vi "Get GPS Data.vi"(8 "error in (no error)":errorcluster, 10 "sensor data":string, 11 "previous partial sentence":string) -> (0 "error out":errorcluster, 2 "GPS data":T1 {"oldest read timestamp" format="%^<%.3X\n%x>T"}, 3 "remaining partial sentence":string)   [LabVIEW 2011, in "u-blox 5 Series.lvlib"]
doc: "Parses <B>instrument data</B> in the NMEA format from GPS devices and returns common <B>GPS data</B>, such as the latitude and longitude of a fix."
uses:
  u-blox 5 Series.lvlib
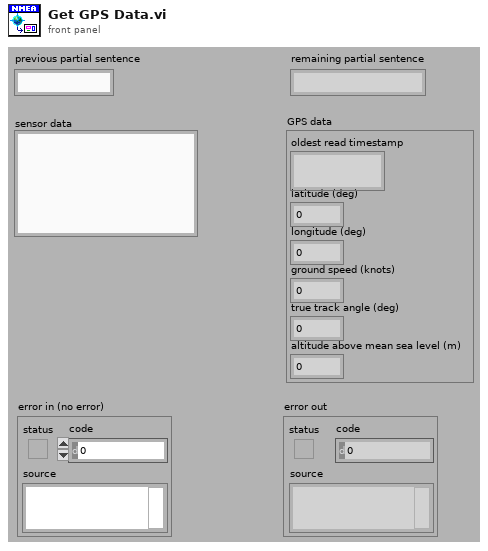
[diagram p1: front panel]
types:
  T1 = cluster{"oldest read timestamp":timestamp, "latitude (deg)":dbl, "longitude (deg)":dbl, "ground speed (knots)":dbl, "true track angle (deg)":dbl, "altitude above mean sea level (m)":dbl}
  T2 = cluster{"oldest read timestamp":timestamp, "latitude":dbl, "longitude":dbl, "speed over ground (knots)":dbl, "true track angle (deg)":dbl, "altitude above mean sea level":dbl}
  T3 = cluster{"Oldest Read Timestamp":timestamp, "Latitude":dbl, "Longitude":dbl, "Speed over Ground (Knots)":dbl, "True Track Angle (Deg)":dbl, "Altitude Above Mean Sea Level":dbl}
  T4 = typedef "u-blox 5 Series.lvlib/RMC Data.ctl" = cluster{"time of fix":cluster{"included?":bool, "time":timestamp}, "status":cluster{"included?":bool, "value":u16}, "latitude":cluster{"included?":bool, "latitude (deg)":dbl}, "longitude":cluster{"included?":bool, "longitude (deg)":dbl}, "ground speed":cluster{"included?":bool, "speed (knots)":dbl}, "true track angle":cluster{"included?":bool, "angle (deg)":dbl}, "magnetic variation":cluster{"included?":bool, "variation (deg)":dbl}, "type of fix":cluster{"included?":bool, "mode":u16}}
  T5 = typedef "u-blox 5 Series.lvlib/GGA Data.ctl" = cluster{"time of fix":cluster{"included?":bool, "time":timestamp}, "latitude":cluster{"included?":bool, "latitude (deg)":dbl}, "longitude":cluster{"included?":bool, "longitude (deg)":dbl}, "fix quality":cluster{"included?":bool, "quality":u16}, "number of satellites in view":cluster{"included?":bool, "number of satellites":i8}, "horizontal dilution of precision":cluster{"included?":bool, "horizontal DOP":dbl}, "altitude above mean sea level":cluster{"included?":bool, "altitude (m)":dbl}, "height of geoid above WGS84":cluster{"included?":bool, "height of geoid (m)":dbl}, "time since last DGPS update":cluster{"included?":bool, "time (s)":dbl}, "DGPS station ID number":cluster{"included?":bool, "station ID number":dbl}}
  T6 = typedef "u-blox 5 Series.lvlib/GLL Data.ctl" = cluster{"latitude":cluster{"included?":bool, "latitude (deg)":dbl}, "longitude":cluster{"included?":bool, "longitude (deg)":dbl}, "time of fix":cluster{"included?":bool, "time":timestamp}, "status":cluster{"included?":bool, "value":u16}, "type of fix":cluster{"included?":bool, "mode":u16}}
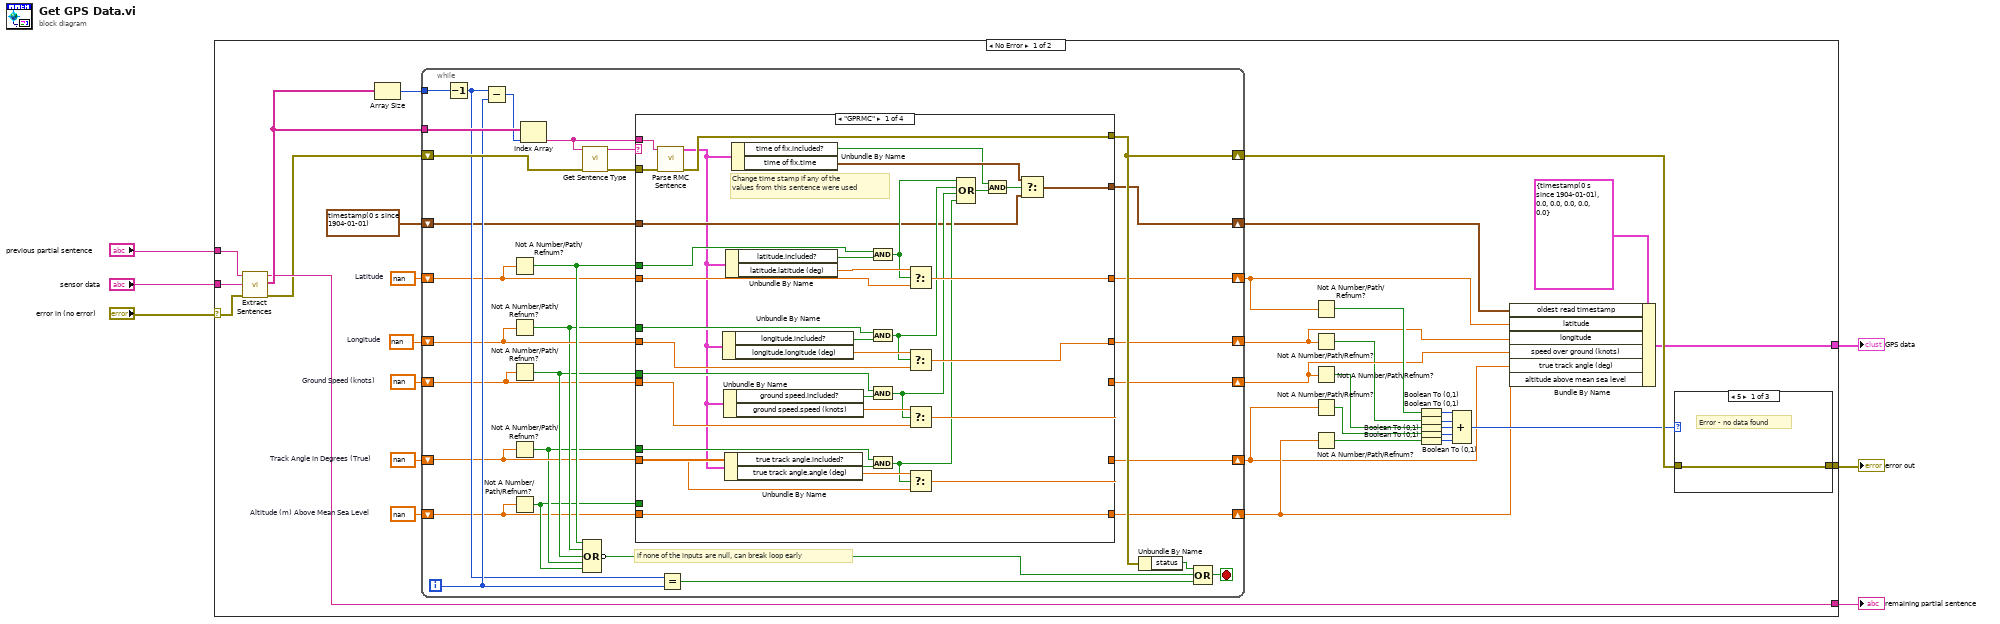
[diagram p0: block diagram]
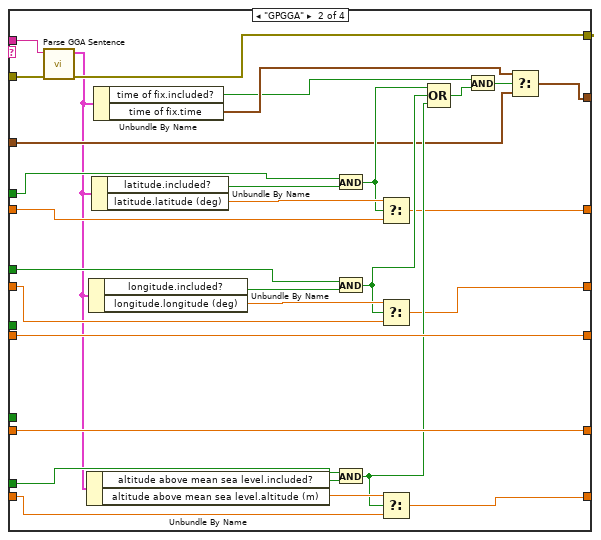
[diagram p4: hidden frame]
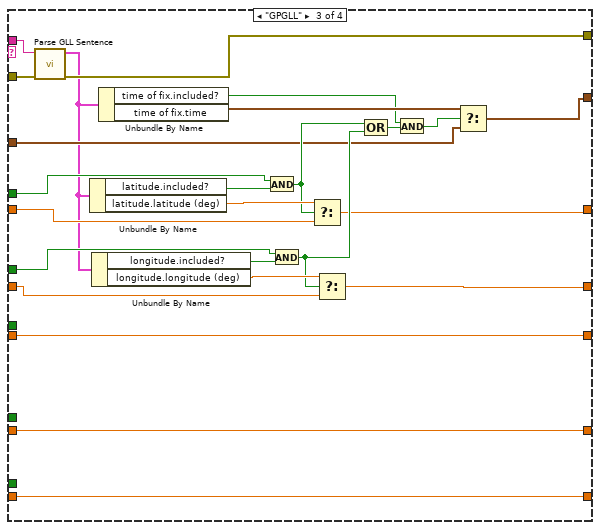
[diagram p5: hidden frame]
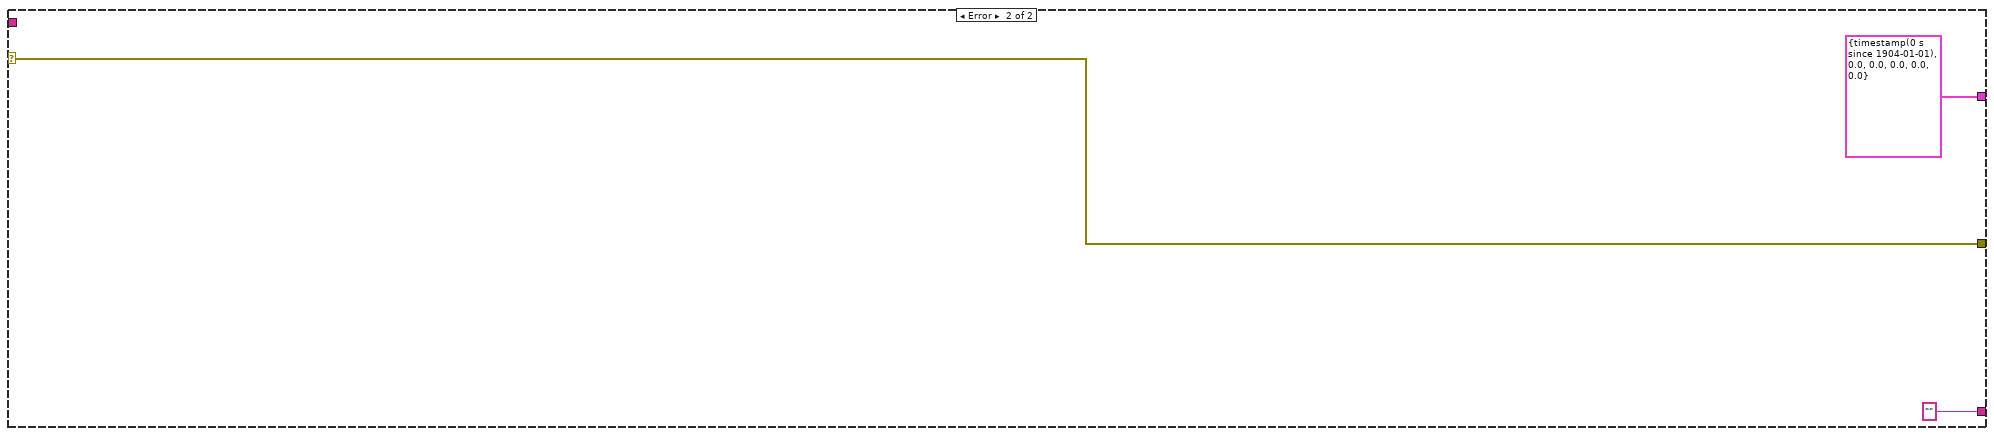
[diagram p7: hidden frame]
diagram:
  n1 = case shown="No Error" "error in (no error)" {
    selector: "error in (no error)" -> [w17 w174]
    tunnel: [w38 w174] -> w5
    tunnel: "sensor data" -> [w26 _]
    tunnel: "previous partial sentence" -> [w25 _]
    tunnel: [w24 T3 {"Oldest Read Timestamp"=timestamp(0 s since 1904-01-01), "Latitude"=0.0, "Longitude"=0.0, "Speed over Ground (Knots)"=0.0, "True Track Angle (Deg)"=0.0, "Altitude Above Mean Sea Level"=0.0} ("GPS Data")] -> w2
    tunnel: [w18 "" ("After Last Sentence")] -> w1
    frame No Error {
      w31 = nan  # Altitude (m) Above Mean Sea Level
      w32 = nan  # Track Angle in Degrees (True)
      w29 = nan  # Ground Speed (knots)
      w33 = nan  # Longitude
      w34 = nan  # Latitude
      n2 = call "Extract Sentences.vi"("error in (no error)"=w17, "sensor data"=w26, "previous partial sentence"=w25) -> ("error out"=w16:errorcluster, "complete sentences"=w37:string[], "remaining partial sentence"=w18:string)  [unwired: 4 in, 2 out]
      n3 = Array Size(array=w37) -> (size(s)=w36:i32)
      n4 = while {
        tunnel: w37 -> [w73]
        shift-right: [w69] -> w39
        shift-left: w16 -> [w71]
        shift-right: [w63] -> w40
        shift-left: timestamp(0 s since 1904-01-01) ("Time of Fix (UTC)") -> [w56]
        shift-right: [w61] -> w28
        shift-left: w34 -> [w54]
        shift-right: [w60] -> w11
        shift-left: w33 -> [w53]
        shift-right: [w68] -> w13
        shift-left: w32 -> [w49]
        shift-right: [w62] -> w14
        shift-left: w31 -> [w46]
        tunnel: w36 -> [w58]
        shift-right: [w59] -> w12
        shift-left: w29 -> [w50]
        i -> [w66]
        stop <- w74 stop-if-true
        # "if none of the inputs are null, can break loop early"
        n5 = Decrement(x=w58) -> (x-1=w57:i32)
        n6 = Subtract(x=w57, y=w66) -> (x-y=w67:i32)
        n7 = Not A Number/Path/Refnum?(number/path/refnum=w54) -> (NaN/Path/Refnum?=w55:bool)
        n8 = Not A Number/Path/Refnum?(number/path/refnum=w53) -> (NaN/Path/Refnum?=w52:bool)
        n9 = Not A Number/Path/Refnum?(number/path/refnum=w50) -> (NaN/Path/Refnum?=w51:bool)
        n10 = Not A Number/Path/Refnum?(number/path/refnum=w49) -> (NaN/Path/Refnum?=w48:bool)
        n11 = Not A Number/Path/Refnum?(number/path/refnum=w46) -> (NaN/Path/Refnum?=w47:bool)
        n12 = Index Array(array=w73, index=w67) -> (element=w45:string)
        n13 = call "Get Sentence Type.vi"("error in (no error)"=w71, "sentence"=w45) -> ("error out"=w70:errorcluster, "sentence type"=w44:string)  [unwired: 1 in, 7 out]
        n14 = Compound Arithmetic op=OR(w55, w52, w51, w48, w47) -> (invert w64:bool)
        n15 = case shown="\"GPRMC\"" w44 {
          tunnel: w70 -> [w109 w139 w164 w171]
          tunnel: [w108 w137 w162 w171] -> w69
          tunnel: [w102 w138 w163 w170] -> w68
          tunnel: w45 -> [w76 w111 w141 _]
          tunnel: w56 -> [w81 w114 w143 w169]
          tunnel: w54 -> [w88 w119 w150 w167]
          tunnel: w53 -> [w93 w125 w156 w166]
          tunnel: w49 -> [w103 w138 w163 w170]
          tunnel: w46 -> [w107 w133 w161 w168]
          tunnel: w55 -> [w90 w120 w151 _]
          tunnel: w52 -> [w95 w127 w152 _]
          tunnel: w51 -> [w97 _ _ _]
          tunnel: w48 -> [w105 _ _ _]
          tunnel: w47 -> [_ w132 _ _]
          tunnel: [w77 w113 w142 w169] -> w63
          tunnel: [w107 w130 w161 w168] -> w62
          tunnel: [w87 w121 w149 w167] -> w61
          tunnel: [w98 w136 w160 w165] -> w59
          tunnel: [w92 w124 w155 w166] -> w60
          tunnel: w50 -> [w99 w136 w160 w165]
          frame "GPRMC" {
            # "Change time stamp if any of the\nvalues from this sentence were used"
            n16 = call "Parse RMC Sentence.vi"("error in (no error)"=w109, "RMC sentence"=w76) -> ("error out"=w108:errorcluster, "RMC data"=w75:T4)  [unwired: 8 in]
            n17 = Unbundle By Name(w75) -> ("longitude.included?"=w96:bool, "longitude.longitude (deg)"=w94:dbl)
            n18 = Unbundle By Name(w75) -> ("ground speed.included?"=w101:bool, "ground speed.speed (knots)"=w100:dbl)
            n19 = Unbundle By Name(w75) -> ("true track angle.included?"=w106:bool, "true track angle.angle (deg)"=w104:dbl)
            n20 = Unbundle By Name(w75) -> ("latitude.included?"=w91:bool, "latitude.latitude (deg)"=w89:dbl)
            n21 = Unbundle By Name(w75) -> ("time of fix.included?"=w79:bool, "time of fix.time"=w80:timestamp)
            n22 = And(x=w90, y=w91) -> (x .and. y?=w86:bool)
            n23 = And(x=w95, y=w96) -> (x .and. y?=w85:bool)
            n24 = And(x=w97, y=w101) -> (x .and. y?=w84:bool)
            n25 = And(x=w105, y=w106) -> (x .and. y?=w83:bool)
            n26 = Select(t=w89, s=w86, f=w88) -> (s? t:f=w87:dbl)
            n27 = Select(t=w94, s=w85, f=w93) -> (s? t:f=w92:dbl)
            n28 = Select(t=w100, s=w84, f=w99) -> (s? t:f=w98:dbl)
            n29 = Select(t=w104, s=w83, f=w103) -> (s? t:f=w102:dbl)
            n30 = Compound Arithmetic op=OR(w86, w85, w84, w83) -> (w82:bool)
            n31 = And(x=w79, y=w82) -> (x .and. y?=w78:bool)
            n32 = Select(t=w80, s=w78, f=w81) -> (s? t:f=w77:timestamp)
          }
          frame "GPGGA" {
            n33 = call "Parse GGA Sentence.vi"("error in (no error)"=w139, "GGA sentence"=w111) -> ("error out"=w137:errorcluster, "GGA data"=w110:T5)  [unwired: 8 in]
            n34 = Unbundle By Name(w110) -> ("altitude above mean sea level.included?"=w135:bool, "altitude above mean sea level.altitude (m)"=w134:dbl)
            n35 = Unbundle By Name(w110) -> ("longitude.included?"=w129:bool, "longitude.longitude (deg)"=w128:dbl)
            n36 = Unbundle By Name(w110) -> ("latitude.included?"=w123:bool, "latitude.latitude (deg)"=w122:dbl)
            n37 = Unbundle By Name(w110) -> ("time of fix.included?"=w116:bool, "time of fix.time"=w117:timestamp)
            n38 = And(x=w120, y=w123) -> (x .and. y?=w118:bool)
            n39 = And(x=w127, y=w129) -> (x .and. y?=w126:bool)
            n40 = And(x=w132, y=w135) -> (x .and. y?=w131:bool)
            n41 = Select(t=w122, s=w118, f=w119) -> (s? t:f=w121:dbl)
            n42 = Select(t=w128, s=w126, f=w125) -> (s? t:f=w124:dbl)
            n43 = Select(t=w134, s=w131, f=w133) -> (s? t:f=w130:dbl)
            n44 = Compound Arithmetic op=OR(w118, w126, w131) -> (w112:bool)
            n45 = And(x=w116, y=w112) -> (x .and. y?=w115:bool)
            n46 = Select(t=w117, s=w115, f=w114) -> (s? t:f=w113:timestamp)
          }
          frame "GPGLL" {
            n47 = call "Parse GLL Sentence.vi"("error in (no error)"=w164, "GLL sentence"=w141) -> ("error out"=w162:errorcluster, "GLL data"=w140:T6)  [unwired: 8 in]
            n48 = Unbundle By Name(w140) -> ("latitude.included?"=w154:bool, "latitude.latitude (deg)"=w153:dbl)
            n49 = Unbundle By Name(w140) -> ("longitude.included?"=w159:bool, "longitude.longitude (deg)"=w158:dbl)
            n50 = Unbundle By Name(w140) -> ("time of fix.included?"=w146:bool, "time of fix.time"=w147:timestamp)
            n51 = And(x=w151, y=w154) -> (x .and. y?=w148:bool)
            n52 = And(x=w152, y=w159) -> (x .and. y?=w157:bool)
            n53 = Select(t=w153, s=w148, f=w150) -> (s? t:f=w149:dbl)
            n54 = Select(t=w158, s=w157, f=w156) -> (s? t:f=w155:dbl)
            n55 = Compound Arithmetic op=OR(w148, w157) -> (w144:bool)
            n56 = And(x=w146, y=w144) -> (x .and. y?=w145:bool)
            n57 = Select(t=w147, s=w145, f=w143) -> (s? t:f=w142:timestamp)
          }
          frame "", Default {
          }
        }
        n58 = Equal?(x=w57, y=w66) -> (x = y?=w72:bool)
        n59 = Unbundle By Name(w69) -> ("status"=w65:bool)
        n60 = Compound Arithmetic op=OR(w65, w64, w72) -> (w74:bool)
      }
      n61 = Not A Number/Path/Refnum?(number/path/refnum=w28) -> (NaN/Path/Refnum?=w15:bool)
      n62 = Not A Number/Path/Refnum?(number/path/refnum=w11) -> (NaN/Path/Refnum?=w10:bool)
      n63 = Not A Number/Path/Refnum?(number/path/refnum=w12) -> (NaN/Path/Refnum?=w9:bool)
      n64 = Not A Number/Path/Refnum?(number/path/refnum=w13) -> (NaN/Path/Refnum?=w8:bool)
      n65 = Not A Number/Path/Refnum?(number/path/refnum=w14) -> (NaN/Path/Refnum?=w7:bool)
      n66 = Boolean To (0,1)(Boolean=w15) -> (0, 1=w23:i16)
      n67 = Boolean To (0,1)(Boolean=w10) -> (0, 1=w22:i16)
      n68 = Boolean To (0,1)(Boolean=w9) -> (0, 1=w21:i16)
      n69 = Boolean To (0,1)(Boolean=w8) -> (0, 1=w20:i16)
      n70 = Boolean To (0,1)(Boolean=w7) -> (0, 1=w19:i16)
      n71 = Compound Arithmetic op=ADD(w23, w22, w21, w20, w19) -> (w27:i16)
      n72 = Bundle By Name(cluster=T2 {"oldest read timestamp"=timestamp(0 s since 1904-01-01), "latitude"=0.0, "longitude"=0.0, "speed over ground (knots)"=0.0, "true track angle (deg)"=0.0, "altitude above mean sea level"=0.0} ("GPS Data"), "oldest read timestamp"=w40, "latitude"=w28, "longitude"=w11, "speed over ground (knots)"=w12, "true track angle (deg)"=w13, "altitude above mean sea level"=w14) -> (w24:T2)
      n73 = case shown="5" w27 {
        tunnel: w39 -> [w41 w42 w43]
        tunnel: [w41 w42 w43] -> w38
        frame 5 {
          # "Error - no data found"
        }
        frame 1..4 {
          # "Warning - not all data found"
        }
        frame 0, Default {
          # "no error"
        }
      }
    }
    frame Error {
    }
  }
  "error out" <- w5
  "remaining partial sentence" <- w1
  "GPS data" <- w2
